vi "hse-application_GetVersionInfos.vi"(8 "error in":errorcluster) -> (0 "error out":errorcluster, 1 "HSE-LIB Version":string, 2 "Framework Version":string, 3 "Application Version":string, 5 "FPGA Version":string, 7 "RT-App Version":string)   [LabVIEW 2020, in "hse-application.lvclass"]
doc: "Returns the various stored version numbers:\nApplication Version: This project (the built application)\nFramework Version: The HSE UI-Framework (Windows Application Template)\nHSE-LIB Version: The hse-libraries \n\n____\nHAMPEL SOFTWARE ENGINEERING v3.8.0 (2023-12-18 14:41)"
uses:
  hse-application.lvclass
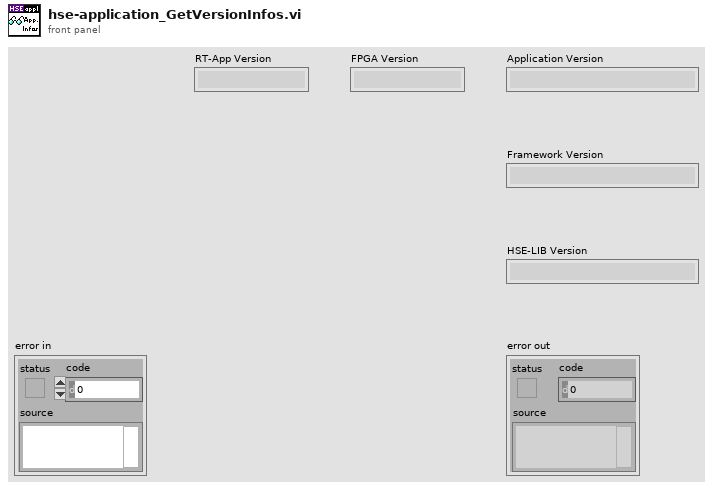
[diagram p1: front panel]
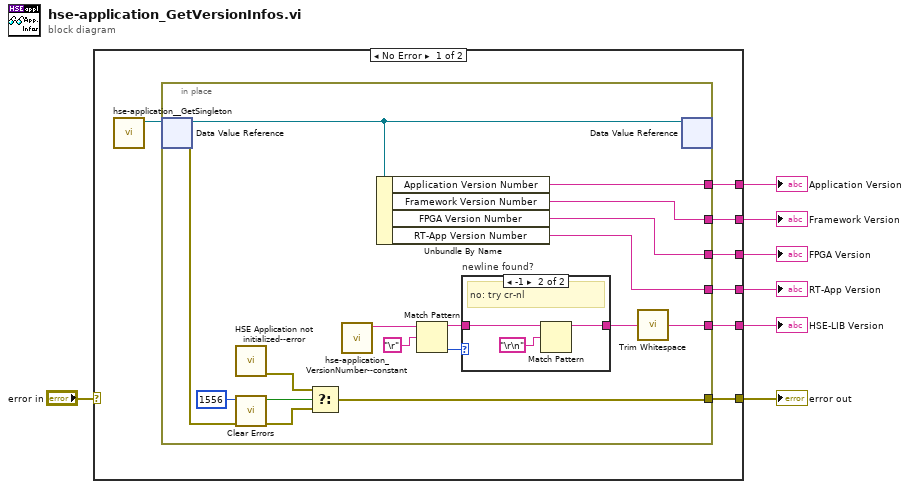
[diagram p0: block diagram]
diagram:
  n1 = case shown="No Error" "error in" {
    selector: "error in" -> [_ w36]
    tunnel: [w14 w36] -> w6
    tunnel: [w13 _] -> w3
    tunnel: [w11 _] -> w4
    tunnel: [w10 _] -> w5
    tunnel: [w9 _] -> w2
    tunnel: [w8 _] -> w1
    frame No Error {
      n2 = call "hse-application__GetSingleton.vi"() -> ("ApplicationClass DVR"=w12:refnum<data-value>)  [unwired: 10 in, 1 out]
      n3 = in-place "In Place Element Structure" {
        in-place-border: [w27] -> w13
        in-place-border: [w28] -> w14
        in-place-border: [w25] -> w11
        in-place-border: [w24] -> w10
        in-place-border: [w23] -> w9
        in-place-border: [w21] -> w8
        n4 = in-place-dvr #1(w12) -> (w26:refnum<class "hse-application.lvclass">, w29:errorcluster)
        n5 = call "HSE Application not initialized--error.vi"() -> ("error out"=w31:errorcluster)  [unwired: 11 in]
        n6 = call <vilib>:"Clear Errors.vi"("error in (no error)"=w29, "specific error code to clear (0: all)"=1556) -> ("error out"=w30:errorcluster, "specific error cleared?"=w15:bool)  [unwired: 4 in]
        n7 = Select(t=w31, s=w15, f=w30) -> (s? t:f=w28:errorcluster)
        n8 = call "hse-application_VersionNumber--constant.vi"() -> ("HSE-Libraries Version Number"=w17:string)  [unwired: 11 in]
        n9 = Unbundle By Name(w26) -> ("Application Version Number"=w24:string, "Framework Version Number"=w25:string, "FPGA Version Number"=w27:string, "RT-App Version Number"=w21:string)
        n10 = Match Pattern(string=w17, regular expression="\r" ("Carriage Return Constant")) -> (before substring=w19:string, offset past match=w20:i32)  [unwired: 1 in, 2 out]
        n11 = case "newline found?" shown="-1" w20 {
          tunnel: w19 -> [w32 w34]
          tunnel: [w32 w33] -> w18
          frame Default {
            # "yes: do nothing"
          }
          frame -1 {
            # "no: try cr-nl"
            n12 = Match Pattern(string=w34, regular expression="\r\n" ("End of Line Constant")) -> (before substring=w33:string)  [unwired: 1 in, 3 out]
          }
        }
        n13 = call <vilib>:"Trim Whitespace.vi"("string"=w18) -> ("trimmed string"=w23:string)  [unwired: 1 in]
        n14 = in-place-dvr #1(w26) -> ()  [unwired: 2 out]
      }
    }
    frame Error {
    }
  }
  "error out" <- w6
  "Application Version" <- w5
  "Framework Version" <- w4
  "FPGA Version" <- w3
  "HSE-LIB Version" <- w2
  "RT-App Version" <- w1
